vi "RxTestExample.vi"() -> ()   [LabVIEW 2015]
uses:
  VISAOperation.ctl
  ONOFF.ctl
panel:
  in  "GenerationConfig":T1={"ExternalAtt"=0.0, "Freq"=5180000000.0, "RxPwr"=-50.0, "PortName"=5, "PacketNumber"=100, "WaveformName(WithType)"="ac80mcs9.tdms"} {"RxPwr" format="%#_13g"; "Freq" format="%#_13g"; "ExternalAtt" format="%#_13g"}
  in  "VISA resource name":refnum<visa-resource-name>="TCPIP0::10.144.41.48::inst0::INSTR"
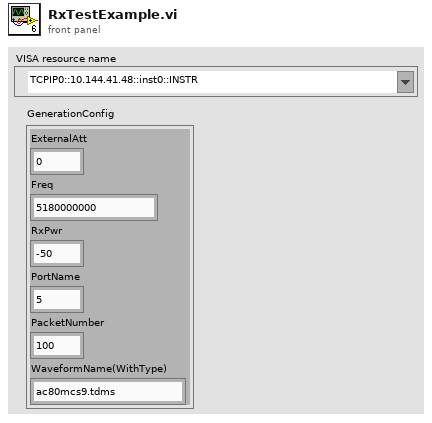
[diagram p1: front panel]
types:
  T1 = cluster{"ExternalAtt":dbl, "Freq":dbl, "RxPwr":dbl, "PortName":i32, "PacketNumber":i32, "WaveformName(WithType)":string}
  T2 = typedef "ONOFF.ctl" = u16
  T3 = typedef "VISAOperation.ctl" = enum16{"RunFile", "OpenDebugPanel", "ReadError", "ReadSTB", "Reset", "Clean", "CloseVISA", "RunCMD", "OpenVISA"}
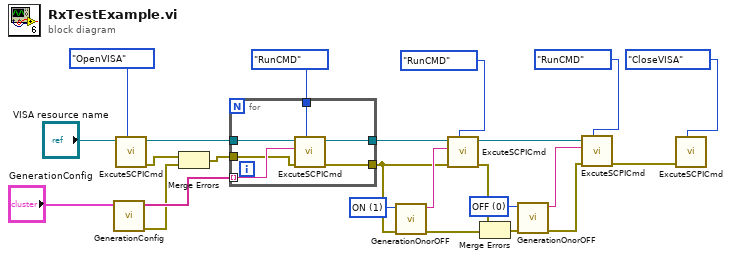
[diagram p0: block diagram]
diagram:
  w1 = T2 0 items=["OFF", "ON"] ("ON/OFF")
  w2 = T2 1 items=["OFF", "ON"] ("ON/OFF")
  n1 = call "GenerationConfig.vi"("GenerationConfig"="GenerationConfig") -> ("error out"=w10:errorcluster, "GenerationConfigCMD"=w19:string[])  [unwired: 9 in]
  n2 = call "ExcuteSCPICmd.vi"("VISAOperation"=VISAOperation."OpenVISA", "VISA resource name"="VISA resource name") -> ("error out"=w11:errorcluster, "reference out"=w22:refnum<visa-resource-name>)  [unwired: 6 in, 2 out]
  n3 = Merge Errors(w11, w10) -> (w9:errorcluster)
  n4 = for {
    tunnel: w22 -> [w30]
    tunnel: VISAOperation."RunCMD" ("VISAOperation") -> [w29]
    tunnel: w19 -> [w28] mode=indexing
    tunnel: [w27] -> w18
    tunnel: w9 -> [w26]
    tunnel: [w25] -> w8
    n5 = call "ExcuteSCPICmd.vi"("VISAOperation"=w29, "error in (no error)"=w26, "Run Command"=w28, "VISA resource name"=w30) -> ("error out"=w25:errorcluster, "reference out"=w27:refnum<visa-resource-name>)  [unwired: 4 in, 2 out]
  }
  n6 = call "GenerationOnorOFF.vi"("error in (no error)"=w8, "ON/OFF"=w2) -> ("error out"=w6:errorcluster, "ON/OFFCMD"=w16:string)  [unwired: 8 in]
  n7 = call "ExcuteSCPICmd.vi"("VISAOperation"=VISAOperation."RunCMD", "error in (no error)"=w8, "Run Command"=w16, "VISA resource name"=w18) -> ("error out"=w5:errorcluster, "reference out"=w14:refnum<visa-resource-name>)  [unwired: 4 in, 2 out]
  n8 = Merge Errors(w5, w6) -> (w7:errorcluster)
  n9 = call "GenerationOnorOFF.vi"("error in (no error)"=w7, "ON/OFF"=w1) -> ("error out"=w4:errorcluster, "ON/OFFCMD"=w13:string)  [unwired: 8 in]
  n10 = call "ExcuteSCPICmd.vi"("VISAOperation"=VISAOperation."RunCMD", "error in (no error)"=w4, "Run Command"=w13, "VISA resource name"=w14) -> ("error out"=w3:errorcluster)  [unwired: 4 in, 3 out]
  n11 = call "ExcuteSCPICmd.vi"("VISAOperation"=VISAOperation."CloseVISA", "error in (no error)"=w3) -> ()  [unwired: 6 in, 4 out]
